vi "Mage Processsing.vi"(0 "Image In":T1, 7 "error in":errorcluster) -> (20 "Image Out":T1, 21 "Matches (Locate Blue)":T2(array[cluster]) {"Bounding Box"."y" format="%.2f"; "Bounding Box"."x" format="%.2f"; "Position"."y" format="%.2f"; "Position"."x" format="%.2f"; "Score" format="%.2f"; "Scale" format="%.2f"; "Angle" format="%.2f"}, 22 "Matches (Locate Green)":T2(array[cluster]) {"Bounding Box"."y" format="%.2f"; "Bounding Box"."x" format="%.2f"; "Position"."y" format="%.2f"; "Position"."x" format="%.2f"; "Score" format="%.2f"; "Scale" format="%.2f"; "Angle" format="%.2f"}, 23 "Matches (Locate Red)":T2(array[cluster]) {"Bounding Box"."y" format="%.2f"; "Bounding Box"."x" format="%.2f"; "Position"."y" format="%.2f"; "Position"."x" format="%.2f"; "Score" format="%.2f"; "Scale" format="%.2f"; "Angle" format="%.2f"}, 27 "error out":errorcluster)   [LabVIEW 2014]
uses:
  <vilib>/vision/Image Controls.llb/IMAQ Image.ctl
  <vilib>/vision/NI_Vision_Development_Module.lvlib
panel:
  out "error out tmp1":errorcluster
  out "error out tmp2":errorcluster
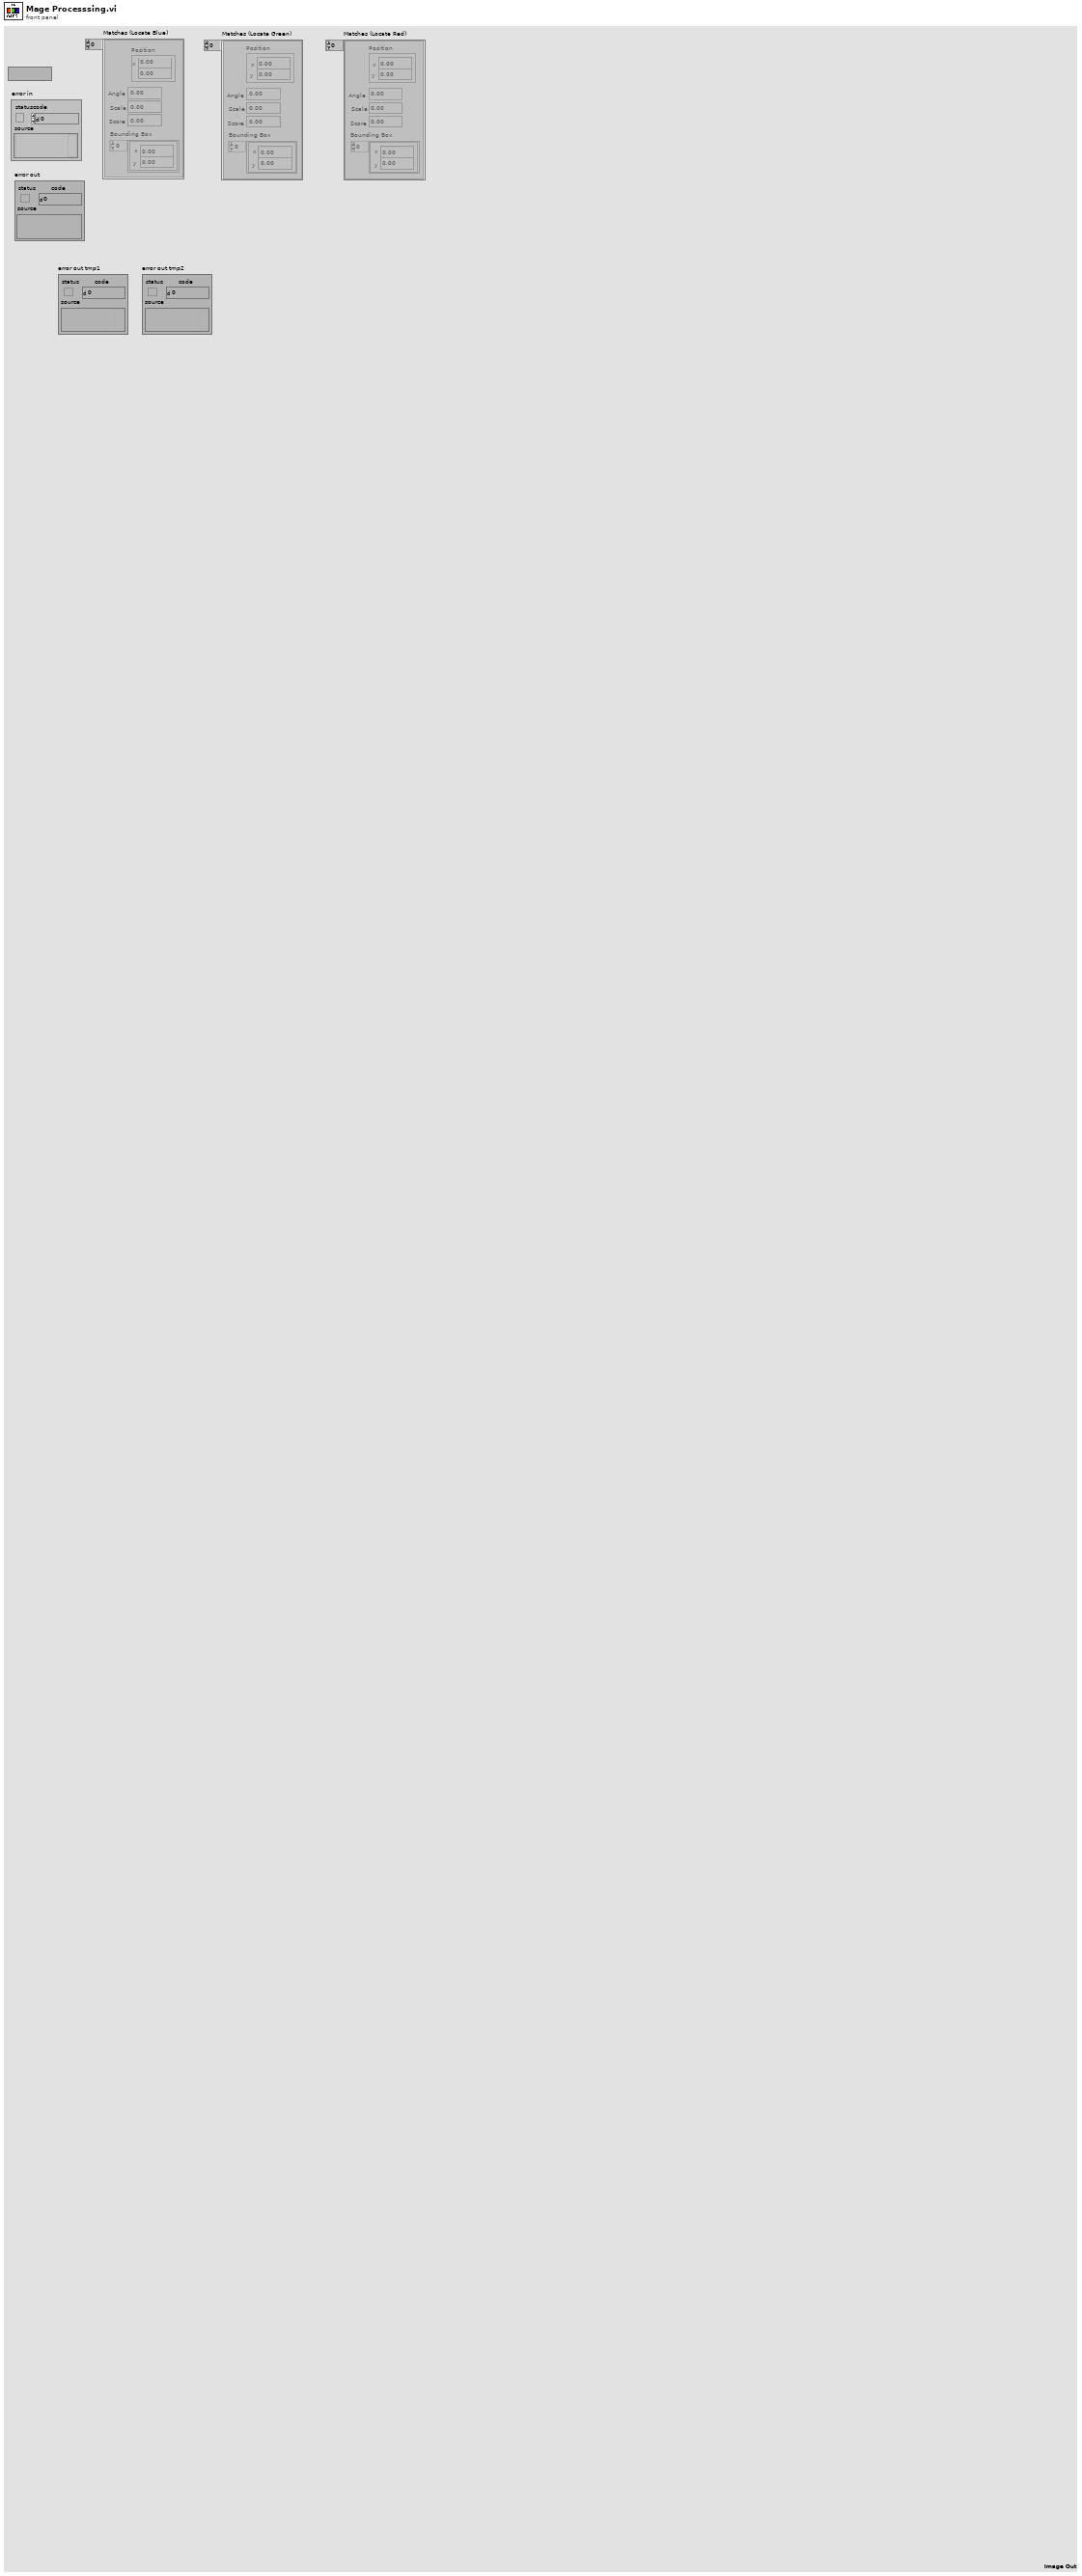
[diagram p1: front panel]
types:
  T1 = typedef "IMAQ Image.ctl" = refnum<image>
  T2 = cluster{"Position":cluster{"x":sgl, "y":sgl}, "Angle":sgl, "Scale":sgl, "Score":sgl, "Bounding Box":cluster{"x":sgl, "y":sgl}[]}[]
  T3 = typedef "Image Type" = u32
  T4 = cluster{"Global Rectangle":i32[], "Contours":cluster{"ID":enum32{"External", "Internal"}, "Type":u32, "Coordinates":i32[]}[]}
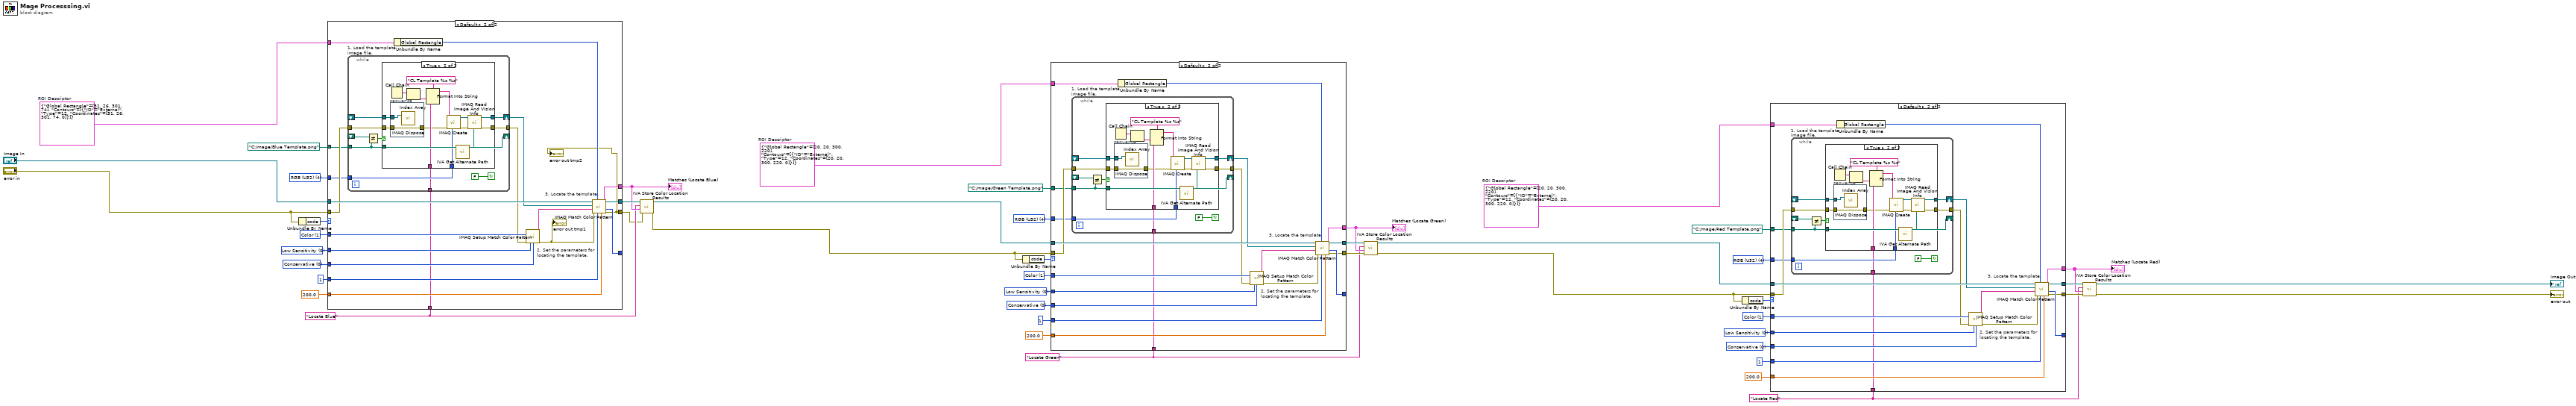
[diagram p0: block diagram]
diagram:
  w7 = "Locate Red" ("Step Name")
  w14 = T3 4 items=["Grayscale (U8)", "Grayscale (I16)", "Grayscale (SGL)", "Complex (CSG)", "RGB (U32)", "HSL (U32)", "RGB (U64)"] ("Image Type")
  w16 = u32 0 items=["Conservative", "Balance", "Aggressive", "Very Aggressive"] ("Search Strategy")
  w17 = u32 0 items=["Low Sensitivity", "Medium Sensitivity", "High Sensitivity"] ("Color Sensitivity")
  w18 = u32 1 items=["Color and Shape", "Color", "Shape"] ("Match Feature Mode")
  w13 = T4 {"Global Rectangle"=[20, 20, 300, 220], "Contours"=[{"ID"=enum."External", "Type"=12, "Coordinates"=[20, 20, 300, 220, 0]}]}  # ROI Descriptor
  w21 = "Locate Green" ("Step Name")
  w29 = T3 4 items=["Grayscale (U8)", "Grayscale (I16)", "Grayscale (SGL)", "Complex (CSG)", "RGB (U32)", "HSL (U32)", "RGB (U64)"] ("Image Type")
  w31 = u32 0 items=["Conservative", "Balance", "Aggressive", "Very Aggressive"] ("Search Strategy")
  w32 = u32 0 items=["Low Sensitivity", "Medium Sensitivity", "High Sensitivity"] ("Color Sensitivity")
  w33 = u32 1 items=["Color and Shape", "Color", "Shape"] ("Match Feature Mode")
  w28 = T4 {"Global Rectangle"=[20, 20, 300, 220], "Contours"=[{"ID"=enum."External", "Type"=12, "Coordinates"=[20, 20, 300, 220, 0]}]}  # ROI Descriptor
  w36 = "Locate Blue" ("Step Name")
  w42 = T3 4 items=["Grayscale (U8)", "Grayscale (I16)", "Grayscale (SGL)", "Complex (CSG)", "RGB (U32)", "HSL (U32)", "RGB (U64)"] ("Image Type")
  w44 = u32 0 items=["Conservative", "Balance", "Aggressive", "Very Aggressive"] ("Search Strategy")
  w45 = u32 0 items=["Low Sensitivity", "Medium Sensitivity", "High Sensitivity"] ("Color Sensitivity")
  w46 = u32 1 items=["Color and Shape", "Color", "Shape"] ("Match Feature Mode")
  w41 = T4 {"Global Rectangle"=[51, 26, 301, 74], "Contours"=[{"ID"=enum."External", "Type"=12, "Coordinates"=[51, 26, 301, 74, 0]}]}  # ROI Descriptor
  n1 = Unbundle By Name("error in") -> ("code"=w39:i32)
  n2 = case shown="Default" w39 {
    tunnel: sgl 200.0 ("Minimum Match Score") -> [_ w67]
    tunnel: 1 ("Number of Matches Requested") -> [_ w66]
    tunnel: [_ w65] -> _
    tunnel: w46 -> [_ w64]
    tunnel: w45 -> [_ w63]
    tunnel: w44 -> [_ w62]
    tunnel: path "C:/mage/Blue Template.png" ("File Path") -> [_ w55]
    tunnel: w42 -> [_ w54]
    tunnel: "error in" -> [_ w56]
    tunnel: w41 -> [_ w60]
    tunnel: [_ w58] -> w37
    tunnel: "Image In" -> [w48 w57]
    tunnel: [w48 w57] -> w38
    tunnel: [_ w49] -> w1
    tunnel: w36 -> [_ w52]
    frame -1074396199, -1074396198 {
      # "Discard Coordinate System Error"
    }
    frame Default {
      # "3. Locate the template."
      # "2. Set the parameters for\nlocating the template."
      n3 = while "1. Load the template image file." {
        shift-right: [w77] -> w53
        shift-left: _ -> [w76]
        tunnel: [w74] -> w51
        tunnel: w56 -> [w73]
        tunnel: w55 -> [w68]
        tunnel: w54 -> [w72]
        tunnel: w52 -> [w71]
        shift-right: [w68] -> _
        shift-left: _ -> [w70]
        stop <- FALSE continue-if-true
        n4 = Not Equal?(x=w70, y=w68) -> (x != y?=w69:bool)
        n5 = case shown="True" w69 {
          tunnel: [w79 w92] -> w77
          tunnel: w76 -> [w79 w84]
          tunnel: [w78 w89] -> w74
          tunnel: w73 -> [w78 w83]
          tunnel: w72 -> [_ w88]
          tunnel: w71 -> [_ w85]
          tunnel: w68 -> [_ w81]
          frame False {
          }
          frame True {
            n6 = Call Chain() -> (call chain=w87:string[])
            n7 = stacked-sequence {
              tunnel: w84 -> [w96]
              tunnel: w83 -> [w95]
              tunnel: [w95] -> w82
              frame #0 {
                n8 = call "IMAQ Dispose"("Image"=w96) -> ()  [unwired: 2 in, 4 out]
              }
            }
            n9 = Index Array(array=w87) -> (element=w86:string)  [unwired: 1 in]
            n10 = Format Into String(format string="CL Template %s %s" ("Image Name"), w86, w85) -> (resulting string=w94:string)  [unwired: 2 in, 1 out]
            n11 = call "IMAQ Create"("Image Name"=w94, "Image Type"=w88, "error in (no error)"=w82) -> ("New Image"=w91:T1, "error out"=w90:errorcluster)  [unwired: 1 in, 1 out]
            n12 = call <vilib>:"IVA Get Alternate Path.vi"("Path In"=w81) -> ("Path Out"=w80:path)  [unwired: 10 out]
            n13 = call "IMAQ Read Image And Vision Info"("File Path"=w80, "error in (no error)"=w90, "Image"=w91) -> ("error out"=w89:errorcluster, "Image Out"=w92:T1)  [unwired: 1 in, 6 out]
          }
        }
      }
      n14 = Unbundle By Name(w60) -> ("Global Rectangle"=w59:i32[])
      n15 = call "IMAQ Setup Match Color Pattern"("Match Feature Mode"=w64, "error in (no error)"=w51, "Color Sensitivity"=w63, "Search Strategy"=w62) -> ("Match Color Pattern Setup Data"=w61:string, "error out"=w50:errorcluster)  [unwired: 5 in, 5 out]
      "error out tmp1" <- w50
      n16 = call "IMAQ Match Color Pattern"("Minimum Match Score"=w67, "Number of Matches Requested"=w66, "Optional Rectangle"=w59, "error in (no error)"=w50, "Match Color Pattern Setup Data"=w61, "Template Image"=w53, "Image"=w57) -> ("error out"=w49:errorcluster, "Number of Matches"=w65:i32, "Matches"=w58:T2)  [unwired: 2 out]
      "error out tmp2" <- w49
    }
  }
  "Matches (Locate Blue)" <- w37
  n17 = call <vilib>:"IVA Store Color Location Results.vi"("error in (no error)"=w1, "Matches"=w37, "Step Name"=w36, "Image in"=w38) -> ("error out"=w2:errorcluster, "Image dup"=w27:T1)  [unwired: 6 out]
  n18 = Unbundle By Name(w2) -> ("code"=w26:i32)
  n19 = case shown="Default" w26 {
    tunnel: sgl 200.0 ("Minimum Match Score") -> [_ w116]
    tunnel: 1 ("Number of Matches Requested") -> [_ w115]
    tunnel: [_ w114] -> _
    tunnel: w33 -> [_ w113]
    tunnel: w32 -> [_ w112]
    tunnel: w31 -> [_ w111]
    tunnel: path "C:/mage/Green Template.png" ("File Path") -> [_ w103]
    tunnel: w29 -> [_ w102]
    tunnel: w2 -> [_ w104]
    tunnel: w28 -> [_ w108]
    tunnel: [_ w106] -> w22
    tunnel: w27 -> [w97 w105]
    tunnel: [w97 w105] -> w23
    tunnel: [_ w99] -> w24
    tunnel: w21 -> [_ w98]
    frame -1074396199, -1074396198 {
      # "Discard Coordinate System Error"
    }
    frame Default {
      # "3. Locate the template."
      # "2. Set the parameters for\nlocating the template."
      n20 = while "1. Load the template image file." {
        shift-right: [w126] -> w101
        shift-left: _ -> [w125]
        tunnel: [w123] -> w100
        tunnel: w104 -> [w122]
        tunnel: w103 -> [w117]
        tunnel: w102 -> [w121]
        tunnel: w98 -> [w120]
        shift-right: [w117] -> _
        shift-left: _ -> [w119]
        stop <- FALSE continue-if-true
        n21 = Not Equal?(x=w119, y=w117) -> (x != y?=w118:bool)
        n22 = case shown="True" w118 {
          tunnel: [w128 w141] -> w126
          tunnel: w125 -> [w128 w133]
          tunnel: [w127 w138] -> w123
          tunnel: w122 -> [w127 w132]
          tunnel: w121 -> [_ w137]
          tunnel: w120 -> [_ w134]
          tunnel: w117 -> [_ w130]
          frame False {
          }
          frame True {
            n23 = Call Chain() -> (call chain=w136:string[])
            n24 = stacked-sequence {
              tunnel: w133 -> [w145]
              tunnel: w132 -> [w144]
              tunnel: [w144] -> w131
              frame #0 {
                n25 = call "IMAQ Dispose"("Image"=w145) -> ()  [unwired: 2 in, 4 out]
              }
            }
            n26 = Index Array(array=w136) -> (element=w135:string)  [unwired: 1 in]
            n27 = Format Into String(format string="CL Template %s %s" ("Image Name"), w135, w134) -> (resulting string=w143:string)  [unwired: 2 in, 1 out]
            n28 = call "IMAQ Create"("Image Name"=w143, "Image Type"=w137, "error in (no error)"=w131) -> ("New Image"=w140:T1, "error out"=w139:errorcluster)  [unwired: 1 in, 1 out]
            n29 = call <vilib>:"IVA Get Alternate Path.vi"("Path In"=w130) -> ("Path Out"=w129:path)  [unwired: 10 out]
            n30 = call "IMAQ Read Image And Vision Info"("File Path"=w129, "error in (no error)"=w139, "Image"=w140) -> ("error out"=w138:errorcluster, "Image Out"=w141:T1)  [unwired: 1 in, 6 out]
          }
        }
      }
      n31 = Unbundle By Name(w108) -> ("Global Rectangle"=w107:i32[])
      n32 = call "IMAQ Setup Match Color Pattern"("Match Feature Mode"=w113, "error in (no error)"=w100, "Color Sensitivity"=w112, "Search Strategy"=w111) -> ("Match Color Pattern Setup Data"=w110:string, "error out"=w109:errorcluster)  [unwired: 5 in, 5 out]
      n33 = call "IMAQ Match Color Pattern"("Minimum Match Score"=w116, "Number of Matches Requested"=w115, "Optional Rectangle"=w107, "error in (no error)"=w109, "Match Color Pattern Setup Data"=w110, "Template Image"=w101, "Image"=w105) -> ("error out"=w99:errorcluster, "Number of Matches"=w114:i32, "Matches"=w106:T2)  [unwired: 2 out]
    }
  }
  "Matches (Locate Green)" <- w22
  n34 = call <vilib>:"IVA Store Color Location Results.vi"("error in (no error)"=w24, "Matches"=w22, "Step Name"=w21, "Image in"=w23) -> ("error out"=w25:errorcluster, "Image dup"=w12:T1)  [unwired: 6 out]
  n35 = Unbundle By Name(w25) -> ("code"=w11:i32)
  n36 = case shown="Default" w11 {
    tunnel: sgl 200.0 ("Minimum Match Score") -> [_ w165]
    tunnel: 1 ("Number of Matches Requested") -> [_ w164]
    tunnel: [_ w163] -> _
    tunnel: w18 -> [_ w162]
    tunnel: w17 -> [_ w161]
    tunnel: w16 -> [_ w160]
    tunnel: path "C:/mage/Red Template.png" ("File Path") -> [_ w152]
    tunnel: w14 -> [_ w151]
    tunnel: w25 -> [_ w153]
    tunnel: w13 -> [_ w157]
    tunnel: [_ w155] -> w8
    tunnel: w12 -> [w146 w154]
    tunnel: [w146 w154] -> w9
    tunnel: [_ w148] -> w10
    tunnel: w7 -> [_ w147]
    frame -1074396199, -1074396198 {
      # "Discard Coordinate System Error"
    }
    frame Default {
      # "3. Locate the template."
      # "2. Set the parameters for\nlocating the template."
      n37 = while "1. Load the template image file." {
        shift-right: [w175] -> w150
        shift-left: _ -> [w174]
        tunnel: [w172] -> w149
        tunnel: w153 -> [w171]
        tunnel: w152 -> [w166]
        tunnel: w151 -> [w170]
        tunnel: w147 -> [w169]
        shift-right: [w166] -> _
        shift-left: _ -> [w168]
        stop <- FALSE continue-if-true
        n38 = Not Equal?(x=w168, y=w166) -> (x != y?=w167:bool)
        n39 = case shown="True" w167 {
          tunnel: [w177 w190] -> w175
          tunnel: w174 -> [w177 w182]
          tunnel: [w176 w187] -> w172
          tunnel: w171 -> [w176 w181]
          tunnel: w170 -> [_ w186]
          tunnel: w169 -> [_ w183]
          tunnel: w166 -> [_ w179]
          frame False {
          }
          frame True {
            n40 = Call Chain() -> (call chain=w185:string[])
            n41 = stacked-sequence {
              tunnel: w182 -> [w194]
              tunnel: w181 -> [w193]
              tunnel: [w193] -> w180
              frame #0 {
                n42 = call "IMAQ Dispose"("Image"=w194) -> ()  [unwired: 2 in, 4 out]
              }
            }
            n43 = Index Array(array=w185) -> (element=w184:string)  [unwired: 1 in]
            n44 = Format Into String(format string="CL Template %s %s" ("Image Name"), w184, w183) -> (resulting string=w192:string)  [unwired: 2 in, 1 out]
            n45 = call "IMAQ Create"("Image Name"=w192, "Image Type"=w186, "error in (no error)"=w180) -> ("New Image"=w189:T1, "error out"=w188:errorcluster)  [unwired: 1 in, 1 out]
            n46 = call <vilib>:"IVA Get Alternate Path.vi"("Path In"=w179) -> ("Path Out"=w178:path)  [unwired: 10 out]
            n47 = call "IMAQ Read Image And Vision Info"("File Path"=w178, "error in (no error)"=w188, "Image"=w189) -> ("error out"=w187:errorcluster, "Image Out"=w190:T1)  [unwired: 1 in, 6 out]
          }
        }
      }
      n48 = Unbundle By Name(w157) -> ("Global Rectangle"=w156:i32[])
      n49 = call "IMAQ Setup Match Color Pattern"("Match Feature Mode"=w162, "error in (no error)"=w149, "Color Sensitivity"=w161, "Search Strategy"=w160) -> ("Match Color Pattern Setup Data"=w159:string, "error out"=w158:errorcluster)  [unwired: 5 in, 5 out]
      n50 = call "IMAQ Match Color Pattern"("Minimum Match Score"=w165, "Number of Matches Requested"=w164, "Optional Rectangle"=w156, "error in (no error)"=w158, "Match Color Pattern Setup Data"=w159, "Template Image"=w150, "Image"=w154) -> ("error out"=w148:errorcluster, "Number of Matches"=w163:i32, "Matches"=w155:T2)  [unwired: 2 out]
    }
  }
  "Matches (Locate Red)" <- w8
  n51 = call <vilib>:"IVA Store Color Location Results.vi"("error in (no error)"=w10, "Matches"=w8, "Step Name"=w7, "Image in"=w9) -> ("error out"=→"error out":errorcluster, "Image dup"=→"Image Out":T1)  [unwired: 6 out]
